vi "Add Digital Command.vi"(8 "error in (no error)":errorcluster, 10 "Command":T1, 11 "Iteration Actions in":refnum<class "Iteration Actions.lvclass">) -> (0 "error out":errorcluster, 3 "Iteration Actions out":refnum<class "Iteration Actions.lvclass">)   [LabVIEW 2020, in "VolatusSeq.lvlib" / "Iteration Actions.lvclass"]
uses:
  Iteration Actions.lvclass
  Command.ctl
  Volatus/MessageQ/MessageQ.lvclass
  Format String/Format String.lvclass
  VolatusSeqConfig/Command Type.ctl
  messages/CmdDigital/Data.ctl
  messages/CmdAnalog/Data.ctl
  Send Type.ctl
  lv-vecto/Vecto/Channel DBL/Channel DBL.lvclass
  Iteration Actions.lvclass/Iteration Actions.ctl
  <vilib>/Utility/miscctls.llb/LVMapReplaceAction.ctl
  messages/CmdDigitalMultiple/Class/Msg.lvclass/Msg.ctl
  messages/CmdDigitalMultiple/Class/Msg.lvclass
  messages/CmdDigital/CmdDigital.lvlib
  VolatusSeqConfig/VolatusSeqConfig.lvlib
  messages/CmdAnalog/CmdAnalog.lvlib
  VolatusSeq.lvlib
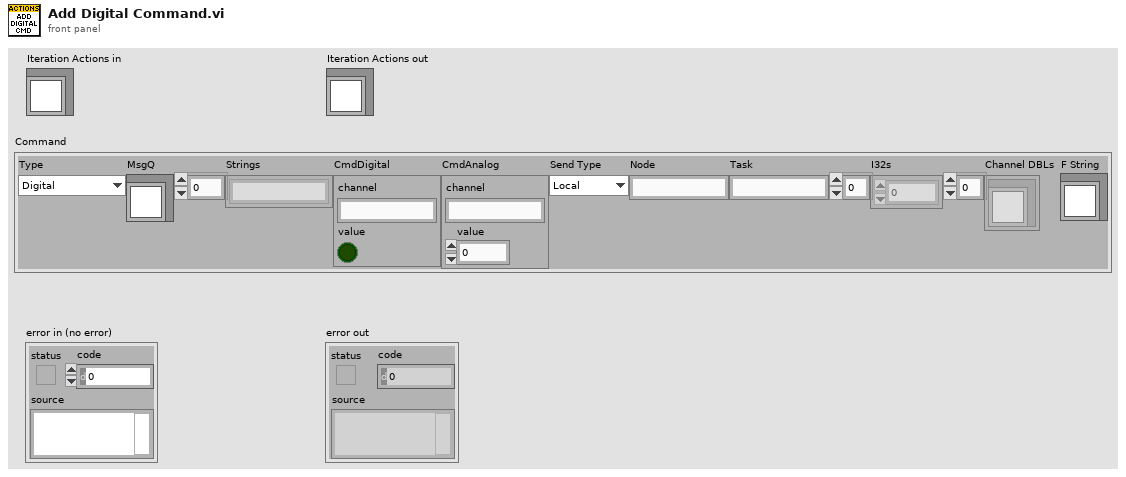
[diagram p1: front panel]
types:
  T1 = typedef "VolatusSeq.lvlib/Command.ctl" = cluster{"Type":T2, "MsgQ":refnum<class "MessageQ.lvclass">, "Strings":string[], "CmdDigital":T3, "CmdAnalog":T4, "Send Type":T5, "Node":string, "Task":string, "I32s":i32[], "Channel DBLs":refnum<class "Channel DBL.lvclass">[], "F String":refnum<class "Format String.lvclass">}
  T2 = typedef "VolatusSeqConfig.lvlib/Command Type.ctl" = enum16{"Digital", "Numeric", "Transition", "Stop", "StartLog", "StopLog", "Start", "Event", "Error", "HTTP", "ResetVar", "IncVar", "DecVar", "SaveVar", "LoadVar", "AddVar", "SubVar", "SetVar", "AddToVar"}
  T3 = typedef "CmdDigital.lvlib/Data.ctl" = cluster{"channel":string, "value":bool}
  T4 = typedef "CmdAnalog.lvlib/Data.ctl" = cluster{"channel":string, "value":dbl}
  T5 = typedef "VolatusSeq.lvlib/Send Type.ctl" = enum16{"Local", "Remote"}
  T6 = typedef "LVMapReplaceAction.ctl" = enum32{"Modify Entry only if found", "Add or Modify Entry", "Delete Entry"}
  T7 = typedef "CmdDigitalMultiple.lvlib/Data.ctl" = cluster{"values":T3[]}
  T8 = typedef "VolatusSeq.lvlib/Remote Digital.ctl" = cluster{"Node":string, "Cmd":T7}
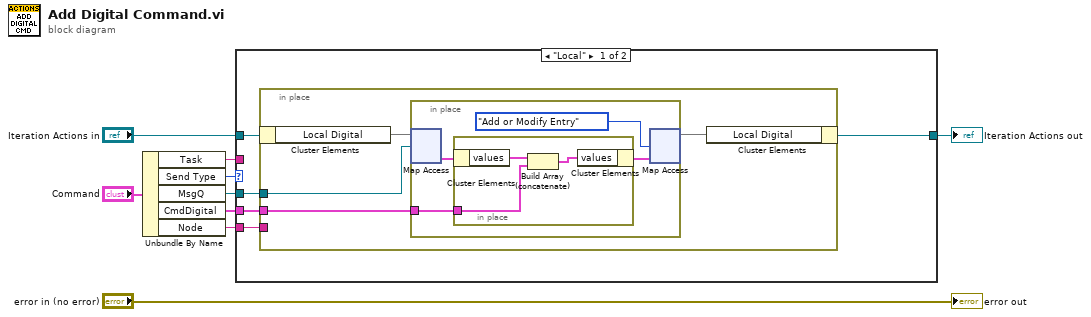
[diagram p0: block diagram]
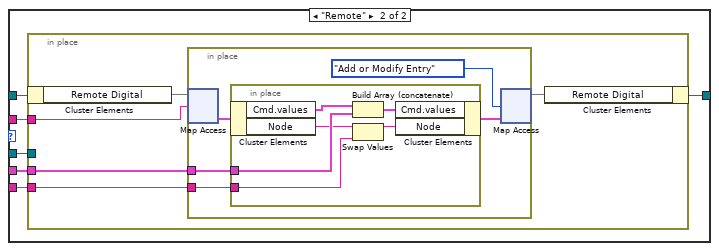
[diagram p2: hidden frame]
diagram:
  n1 = Unbundle By Name("Command") -> ("Task"=w2:string, "Send Type"=w5:T5, "MsgQ"=w4:refnum<class "MessageQ.lvclass">, "CmdDigital"=w3:T3, "Node"=w1:string)
  n2 = case shown="\"Local\"" w5 {
    tunnel: "Iteration Actions in" -> [w14 w31]
    tunnel: [w13 w30] -> w7
    tunnel: w4 -> [w11 w28]
    tunnel: w3 -> [w12 w29]
    tunnel: w2 -> [_ w26]
    tunnel: w1 -> [w10 w27]
    frame "Local" {
      n3 = in-place {
        in-place-border: w12 -> [w15]
        in-place-border: w11 -> [w16]
        in-place-border: w10 -> [_]
        n4 = in-place-cluster #1(w14) -> ("Local Digital"=w18:map{refnum<class "MessageQ.lvclass">, T7})
        n5 = in-place {
          in-place-border: w15 -> [w19]
          n6 = in-place-map #2(w18, w16) -> (w21:T7)  [unwired: 1 in, 1 out]
          n7 = in-place {
            in-place-border: w19 -> [w23]
            n8 = in-place-cluster #3(w21) -> ("values"=w25:T3[])
            n9 = Build Array (concatenate)(w25, w23) -> (w24:T3[])
            n10 = in-place-cluster #3("values"=w24) -> (w20:T7)
          }
          n11 = in-place-map #2(w20, LVMapReplaceAction."Add or Modify Entry" ("action")) -> (w17:map{refnum<class "MessageQ.lvclass">, T7})  [unwired: 2 out]
        }
        n12 = in-place-cluster #1("Local Digital"=w17) -> (w13:refnum<class "Iteration Actions.lvclass">)
      }
    }
    frame "Remote" {
      n13 = in-place {
        in-place-border: w29 -> [w34]
        in-place-border: w28 -> [_]
        in-place-border: w27 -> [w32]
        in-place-border: w26 -> [w33]
        n14 = in-place-cluster #4(w31) -> ("Remote Digital"=w36:map{string, T8})
        n15 = in-place {
          in-place-border: w34 -> [w38]
          in-place-border: w32 -> [w37]
          n16 = in-place-map #5(w36, w33) -> (w40:T8)  [unwired: 1 in, 1 out]
          n17 = in-place {
            in-place-border: w38 -> [w46]
            in-place-border: w37 -> [w43]
            n18 = in-place-cluster #6(w40) -> ("Cmd.values"=w47:T3[], "Node"=w44:string)
            n19 = Build Array (concatenate)(w47, w46) -> (w45:T3[])
            n20 = Swap Values(12:w44, 14:w43) -> (1:w42:string)  [unwired: 1 in, 1 out]
            n21 = in-place-cluster #6("Cmd.values"=w45, "Node"=w42) -> (w39:T8)
          }
          n22 = in-place-map #5(w39, LVMapReplaceAction."Add or Modify Entry" ("action")) -> (w35:map{string, T8})  [unwired: 2 out]
        }
        n23 = in-place-cluster #4("Remote Digital"=w35) -> (w30:refnum<class "Iteration Actions.lvclass">)
      }
    }
  }
  "Iteration Actions out" <- w7
  "error out" <- "error in (no error)"
